vi "filter.insert.order.vi"(11 "filter.data in":T1 {"memory.command"."order.slot.value"."Quantity" format="%016x"; "memory.command"."order.slot.value"."OrderId" format="%016x"; "memory.command"."ticker.slot.value"."Symbol" format="%016x"; "Scratch"."OrderId" format="%016x"}) -> (3 "filter.data out":T1 {"memory.command"."order.slot.value"."Quantity" format="%016x"; "memory.command"."order.slot.value"."OrderId" format="%016x"; "memory.command"."ticker.slot.value"."Symbol" format="%016x"; "Scratch"."OrderId" format="%016x"})   [LabVIEW 2022 SP3]
uses:
  filter.data.ctl
  filter.states.ctl
  filter.debug.ctl
  filter.debug.slot.ctl
  filter.data.scratch.ctl
  arty/orderbook/orderbook.command.ctl
  arty/orderbook/orderbook.command.type.ctl
  filter.memory.command.ctl
  ticker.slot.ctl
  order.slot.ctl
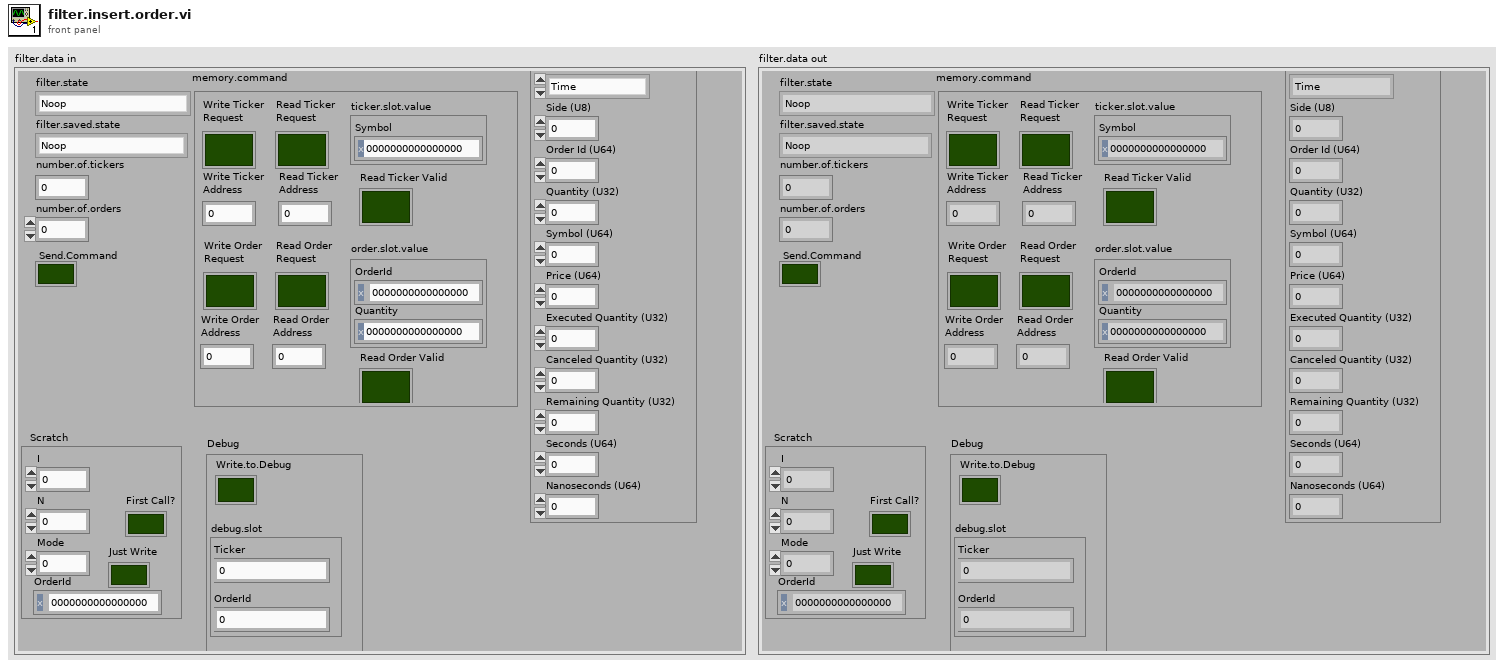
[diagram p1: front panel]
types:
  T1 = typedef "filter.data.ctl" = cluster{"filter.state":T2, "Debug":T3, "number.of.tickers":u32, "number.of.orders":u32, "filter.saved.state":T2, "Scratch":T5, "OrderBook.Command":T6, "Send.Command":bool, "memory.command":T8}
  T2 = typedef "filter.states.ctl" = enum16{"Noop", "Reset", "Debug", "Configuration", "Wait.for.Command", "Filter.Add", "Filter.Other", "Insert.Order", "Delete Order"}
  T3 = typedef "filter.debug.ctl" = cluster{"Write.to.Debug":bool, "debug.slot":T4}
  T4 = typedef "filter.debug.slot.ctl" = cluster{"Ticker":u64, "OrderId":u64}
  T5 = typedef "filter.data.scratch.ctl" = cluster{"I":u32, "N":u32, "Mode":u32, "OrderId":u64, "First Call?":bool, "Just Write":bool}
  T6 = typedef "orderbook.command.ctl" = cluster{"OrderBook Command.Type":T7, "Side (U8)":u8, "Order Id (U64)":u64, "Quantity (U32)":u32, "Symbol (U64)":u64, "Price (U64)":u64, "Executed Quantity (U32)":u32, "Canceled Quantity (U32)":u32, "Remaining Quantity (U32)":u32, "Seconds (U64)":u64, "Nanoseconds (U64)":u64}
  T7 = typedef "orderbook.command.type.ctl" = enum16{"Time", "AddOrder", "OrderExecuted", "OrderExecutedAtPrice", "ReduceSize", "ModifyOrder", "DeleteOrder", "Get.All.Orders", "Get.Top"}
  T8 = typedef "filter.memory.command.ctl" = cluster{"ticker.slot.value":T9, "order.slot.value":T10, "Write Ticker\nAddress":u32, "Write Ticker\nRequest":bool, "Read Ticker\nRequest":bool, "Read Ticker\nAddress":u32, "Read Ticker Valid":bool, "Write Order\nAddress":u32, "Write Order\nRequest":bool, "Read Order\nRequest":bool, "Read Order\nAddress":u32, "Read Order Valid":bool}
  T9 = typedef "ticker.slot.ctl" = cluster{"Symbol":u64}
  T10 = typedef "order.slot.ctl" = cluster{"OrderId":u64, "Quantity":u64}
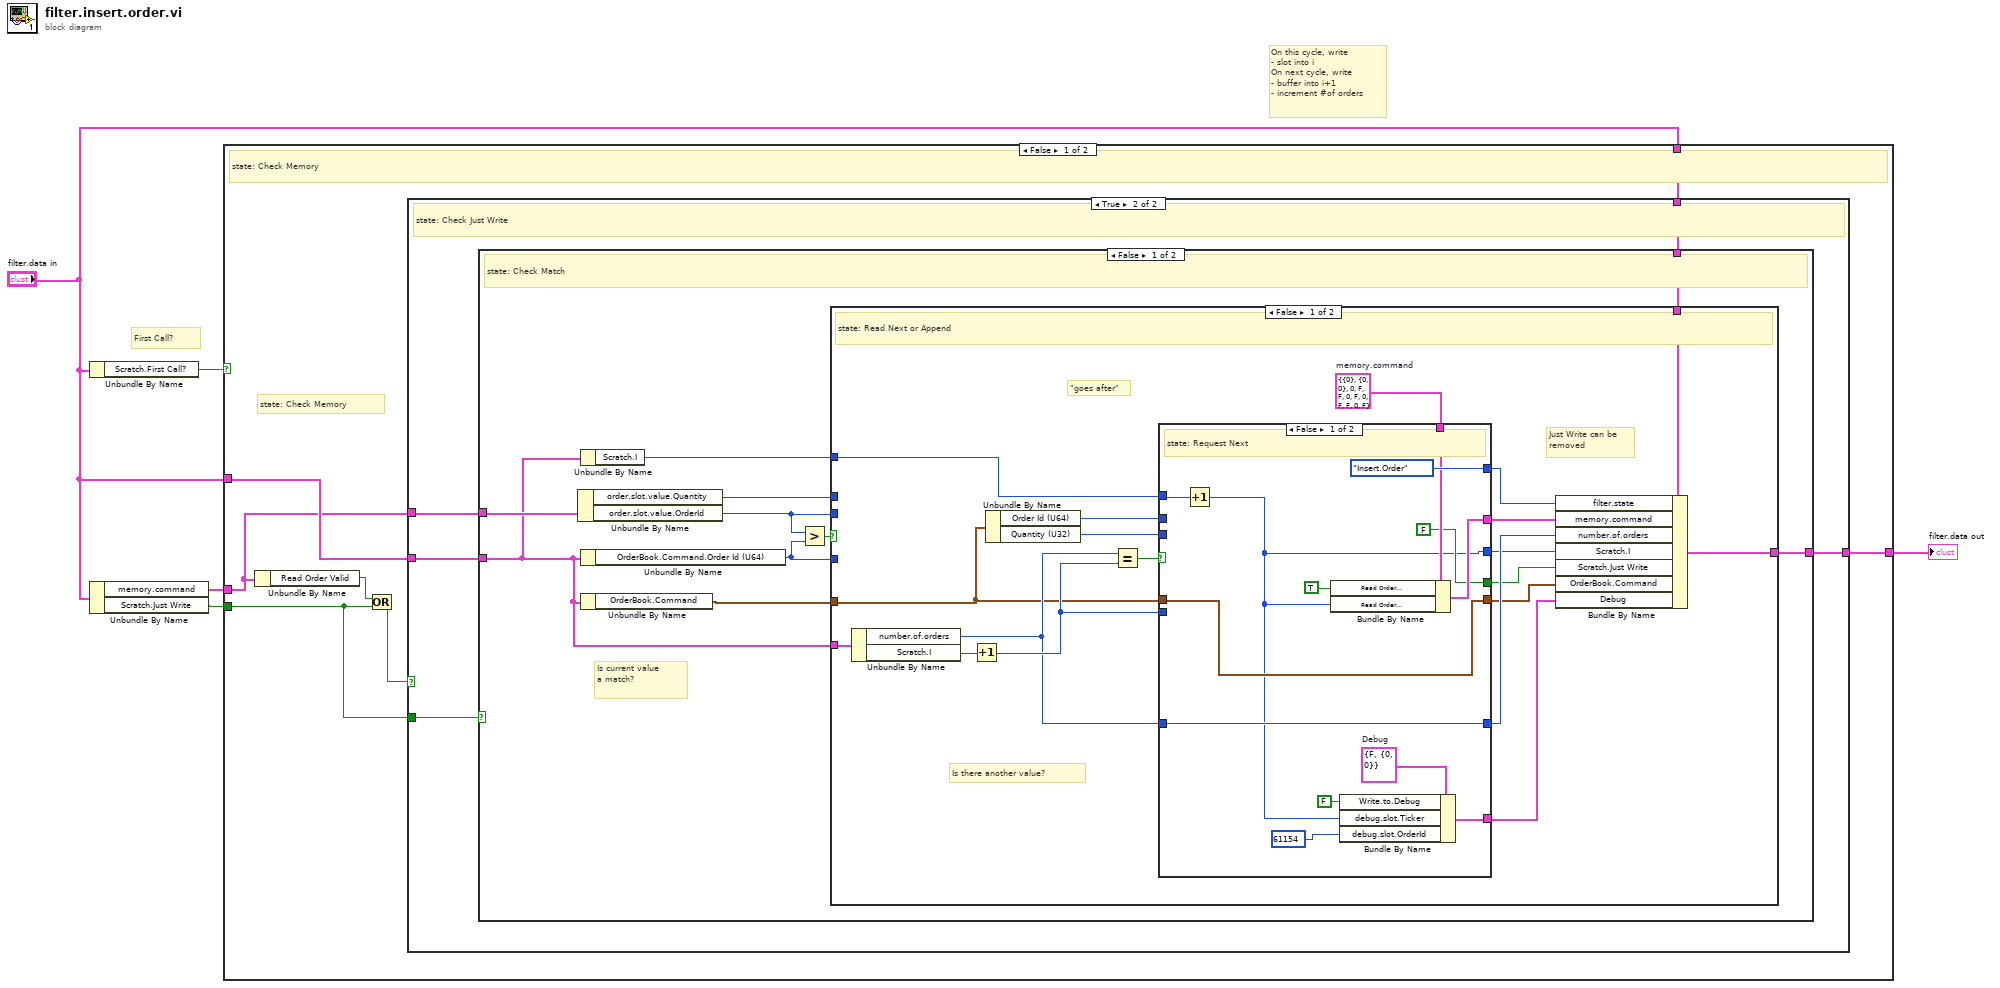
[diagram p0: block diagram]
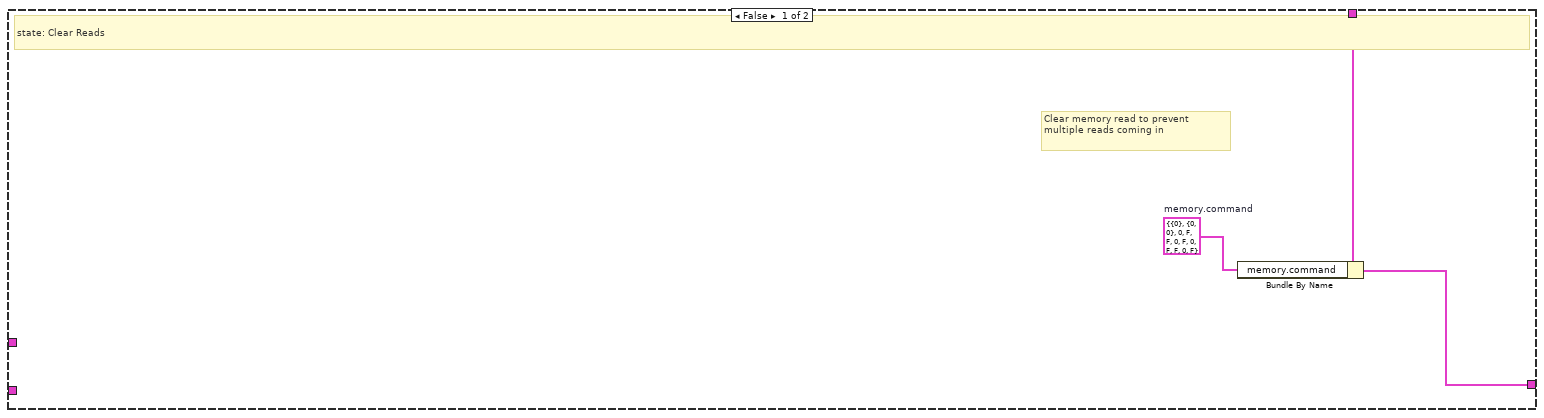
[diagram p2: hidden frame]
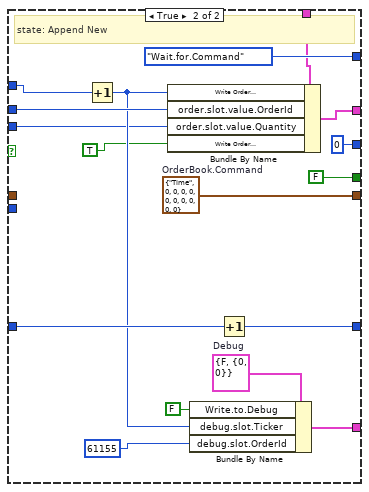
[diagram p3: hidden frame]
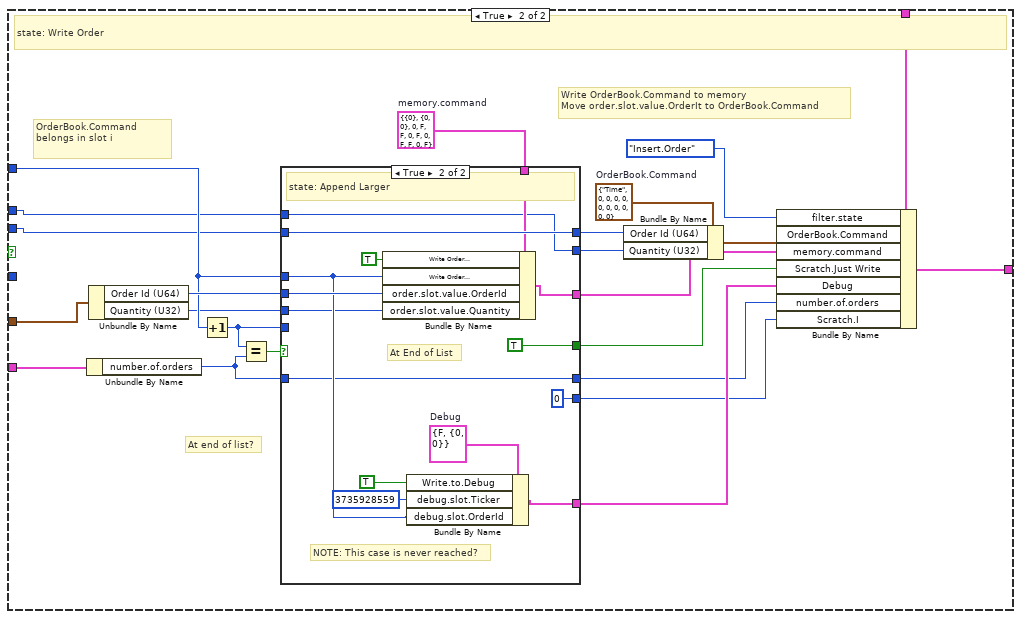
[diagram p4: hidden frame]
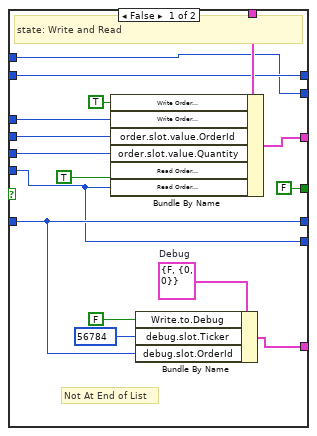
[diagram p5: hidden frame]
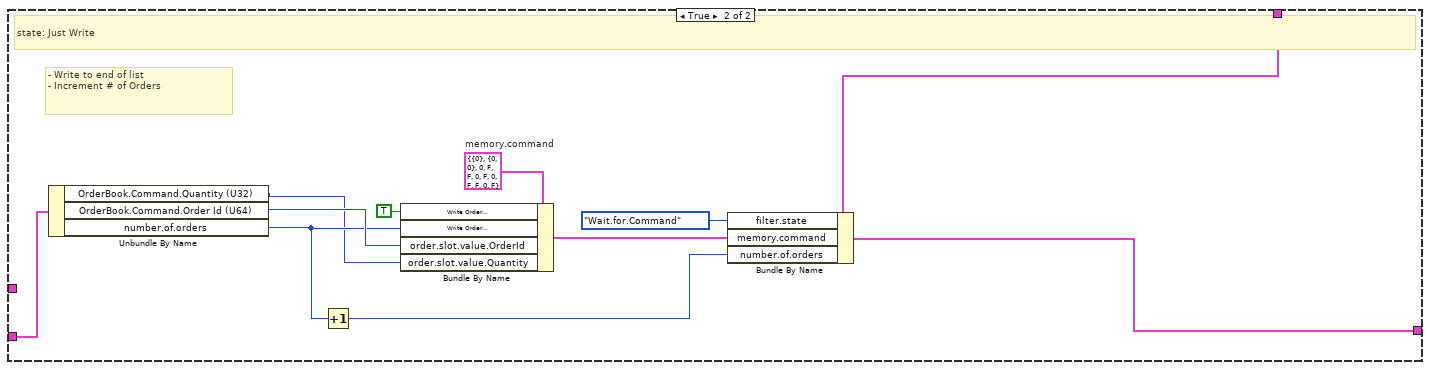
[diagram p6: hidden frame]
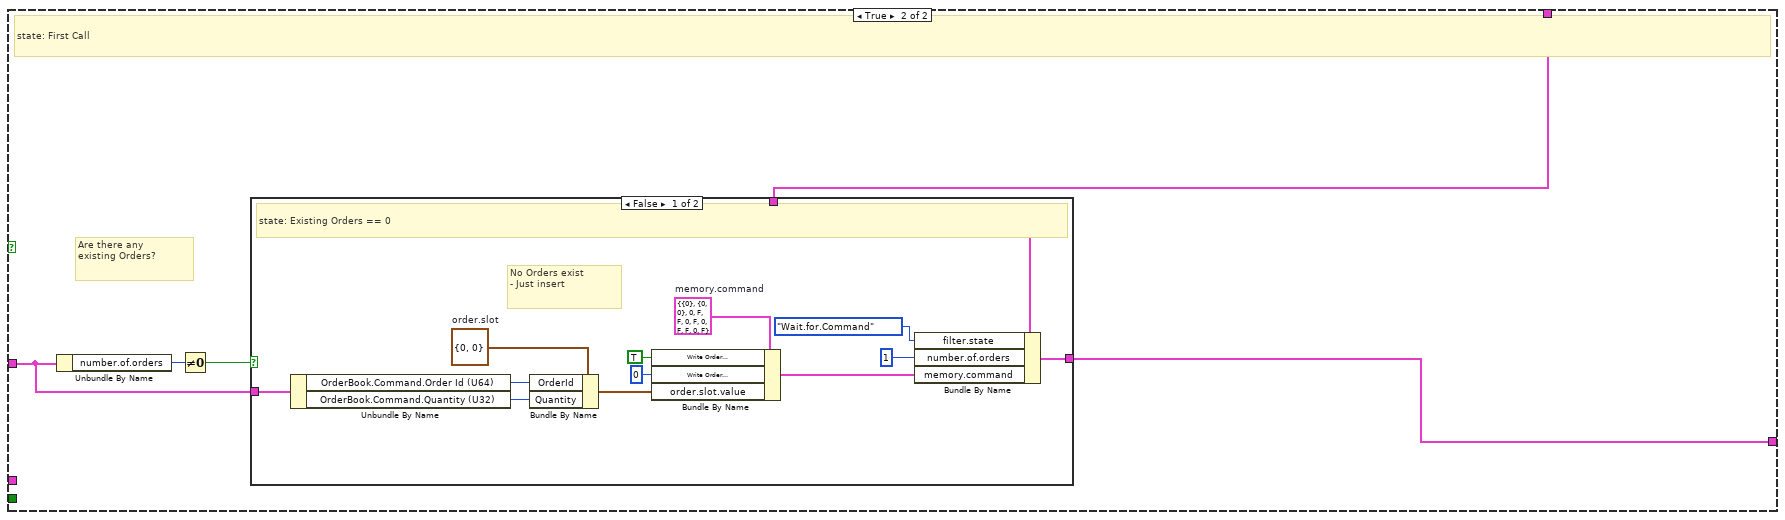
[diagram p7: hidden frame]
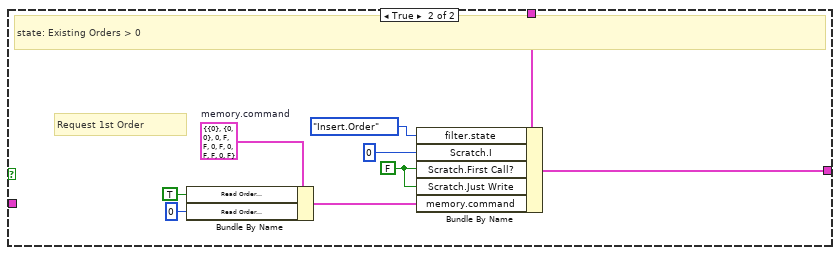
[diagram p8: hidden frame]
diagram:
  # "On this cycle, write\n- slot into i\nOn next cycle, write\n- buffer into i+1\n- increment #of orders"
  # "First Call?"
  n1 = Unbundle By Name("filter.data in") -> ("Scratch.First Call?"=w2:bool)
  n2 = Unbundle By Name("filter.data in") -> ("memory.command"=w4:T8, "Scratch.Just Write"=w1:bool)
  n3 = case shown="False" w2 {
    tunnel: "filter.data in" -> [w11 w147]
    tunnel: [w12 w145] -> w3
    tunnel: w4 -> [w9 _]
    tunnel: "filter.data in" -> [w10 w146]
    tunnel: w1 -> [w6 _]
    frame False {
      # "state: Check Memory"
      # "state: Check Memory"
      n4 = Unbundle By Name(w9) -> ("Read Order Valid"=w8:bool)
      n5 = Or(x=w8, y=w6) -> (x .or. y?=w7:bool)
      n6 = case shown="True" w7 {
        tunnel: [w13 w18] -> w12
        tunnel: w11 -> [w15 w19]
        tunnel: w10 -> [_ w17]
        tunnel: w9 -> [_ w20]
        tunnel: w6 -> [_ w16]
        frame False {
          w14 = T8 {"ticker.slot.value"={"Symbol"=0}, "order.slot.value"={"OrderId"=0, "Quantity"=0}, "Write Ticker\nAddress"=0, "Write Ticker\nRequest"=FALSE, "Read Ticker\nRequest"=FALSE, "Read Ticker\nAddress"=0, "Read Ticker Valid"=FALSE, "Write Order\nAddress"=0, "Write Order\nRequest"=FALSE, "Read Order\nRequest"=FALSE, "Read Order\nAddress"=0, "Read Order Valid"=FALSE}  # memory.command
          # "Clear memory read to prevent\nmultiple reads coming in"
          # "state: Clear Reads"
          n7 = Bundle By Name(cluster=w15, "memory.command"=w14) -> (w13:T1)
        }
        frame True {
          # "state: Check Just Write"
          n8 = case shown="False" w16 {
            tunnel: w20 -> [w30 _]
            tunnel: w19 -> [w28 w141]
            tunnel: [w27 w140] -> w18
            tunnel: w17 -> [w23 w138]
            frame False {
              # "Is current value\na match?"
              # "state: Check Match"
              n9 = Unbundle By Name(w30) -> ("order.slot.value.Quantity"=w21:u64, "order.slot.value.OrderId"=w25:u64)
              n10 = Unbundle By Name(w23) -> ("Scratch.I"=w22:u32)
              n11 = Unbundle By Name(w23) -> ("OrderBook.Command.Order Id (U64)"=w24:u64)
              n12 = Unbundle By Name(w23) -> ("OrderBook.Command"=w26:T6)
              n13 = Greater?(x=w25, y=w24) -> (0:w29:bool)
              n14 = case shown="False" w29 {
                tunnel: w28 -> [w48 w102]
                tunnel: [w49 w100] -> w27
                tunnel: w26 -> [w33 w95]
                tunnel: w23 -> [w47 w92]
                tunnel: w25 -> [_ w87]
                tunnel: w22 -> [w38 w93]
                tunnel: w24 -> [_ _]
                tunnel: w21 -> [_ w80]
                frame False {
                  w40 = T8 {"ticker.slot.value"={"Symbol"=0}, "order.slot.value"={"OrderId"=0, "Quantity"=0}, "Write Ticker\nAddress"=0, "Write Ticker\nRequest"=FALSE, "Read Ticker\nRequest"=FALSE, "Read Ticker\nAddress"=0, "Read Ticker Valid"=FALSE, "Write Order\nAddress"=0, "Write Order\nRequest"=FALSE, "Read Order\nRequest"=FALSE, "Read Order\nAddress"=0, "Read Order Valid"=FALSE}  # memory.command
                  # "Just Write can be\nremoved"
                  # "\"goes after\""
                  # "Is there another value?"
                  # "state: Read Next or Append"
                  n15 = Unbundle By Name(w47) -> ("number.of.orders"=w37:u32, "Scratch.I"=w46:u32)
                  n16 = Increment(x=w46) -> (x+1=w43:u32)
                  n17 = Unbundle By Name(w33) -> ("Order Id (U64)"=w39:u64, "Quantity (U32)"=w31:u32)
                  n18 = Equal?(x=w37, y=w43) -> (x = y?=w44:bool)
                  n19 = case shown="False" w44 {
                    tunnel: [w62 w76] -> w45
                    tunnel: w43 -> [_ _]
                    tunnel: [filter.states."Insert.Order" ("filter.state") filter.states."Wait.for.Command" ("filter.state")] -> w42
                    tunnel: [w58 w72] -> w41
                    tunnel: w40 -> [w59 w78]
                    tunnel: w39 -> [_ w77]
                    tunnel: w38 -> [w51 w75]
                    tunnel: w37 -> [w58 w74]
                    tunnel: [w50 u32 0] -> w36
                    tunnel: [FALSE ("Scratch.Just Write") FALSE ("Scratch.Just Write")] -> w35
                    tunnel: [w56 w70] -> w34
                    tunnel: w33 -> [w56 _]
                    tunnel: [w54 w68] -> w32
                    tunnel: w31 -> [_ w63]
                    frame False {
                      w55 = T3 {"Write.to.Debug"=FALSE, "debug.slot"={"Ticker"=0, "OrderId"=0}}  # Debug
                      # "state: Request Next"
                      n20 = Increment(x=w51) -> (x+1=w50:u32)
                      n21 = Bundle By Name(cluster=w59, "Read Order\nRequest"=TRUE ("Read.Request"), "Read Order\nAddress"=w50) -> (w62:T8)
                      n22 = Bundle By Name(cluster=w55, "Write.to.Debug"=FALSE, "debug.slot.Ticker"=w50, "debug.slot.OrderId"=u64 61154) -> (w54:T3)
                    }
                    frame True {
                      w69 = T3 {"Write.to.Debug"=FALSE, "debug.slot"={"Ticker"=0, "OrderId"=0}}  # Debug
                      w70 = T6 {"OrderBook Command.Type"=enum."Time", "Side (U8)"=0, "Order Id (U64)"=0, "Quantity (U32)"=0, "Symbol (U64)"=0, "Price (U64)"=0, "Executed Quantity (U32)"=0, "Canceled Quantity (U32)"=0, "Remaining Quantity (U32)"=0, "Seconds (U64)"=0, "Nanoseconds (U64)"=0}  # OrderBook.Command
                      # "state: Append New"
                      n23 = Increment(x=w75) -> (x+1=w65:u32)
                      n24 = Bundle By Name(cluster=w78, "Write Order\nAddress"=w65, "order.slot.value.OrderId"=w77, "order.slot.value.Quantity"=w63, "Write Order\nRequest"=TRUE ("Write Order\nRequest")) -> (w76:T8)
                      n25 = Bundle By Name(cluster=w69, "Write.to.Debug"=FALSE, "debug.slot.Ticker"=w65, "debug.slot.OrderId"=u64 61155) -> (w68:T3)
                      n26 = Increment(x=w74) -> (x+1=w72:u32)
                    }
                  }
                  n27 = Bundle By Name(cluster=w48, "filter.state"=w42, "memory.command"=w45, "number.of.orders"=w41, "Scratch.I"=w36, "Scratch.Just Write"=w35, "OrderBook.Command"=w34, "Debug"=w32) -> (w49:T1)
                }
                frame True {
                  w98 = T6 {"OrderBook Command.Type"=enum."Time", "Side (U8)"=0, "Order Id (U64)"=0, "Quantity (U32)"=0, "Symbol (U64)"=0, "Price (U64)"=0, "Executed Quantity (U32)"=0, "Canceled Quantity (U32)"=0, "Remaining Quantity (U32)"=0, "Seconds (U64)"=0, "Nanoseconds (U64)"=0}  # OrderBook.Command
                  w97 = T8 {"ticker.slot.value"={"Symbol"=0}, "order.slot.value"={"OrderId"=0, "Quantity"=0}, "Write Ticker\nAddress"=0, "Write Ticker\nRequest"=FALSE, "Read Ticker\nRequest"=FALSE, "Read Ticker\nAddress"=0, "Read Ticker Valid"=FALSE, "Write Order\nAddress"=0, "Write Order\nRequest"=FALSE, "Read Order\nRequest"=FALSE, "Read Order\nAddress"=0, "Read Order Valid"=FALSE}  # memory.command
                  # "At end of list?"
                  # "Write OrderBook.Command to memory\nMove order.slot.value.OrderIt to OrderBook.Command"
                  # "OrderBook.Command\nbelongs in slot i"
                  # "state: Write Order"
                  n28 = Unbundle By Name(w92) -> ("number.of.orders"=w84:u32)
                  n29 = Unbundle By Name(w95) -> ("Order Id (U64)"=w94:u64, "Quantity (U32)"=w82:u32)
                  n30 = Increment(x=w93) -> (x+1=w91:u32)
                  n31 = Equal?(x=w91, y=w84) -> (x = y?=w90:bool)
                  n32 = case shown="True" w90 {
                    tunnel: w97 -> [w118 w132]
                    tunnel: [w117 w131] -> w96
                    tunnel: w94 -> [w116 w130]
                    tunnel: w93 -> [w113 w123]
                    tunnel: w91 -> [w105 _]
                    tunnel: [w112 w133] -> w89
                    tunnel: w87 -> [w112 w133]
                    tunnel: [FALSE ("Scratch.Just Write") TRUE ("Scratch.Just Write")] -> w88
                    tunnel: [w107 w124] -> w86
                    tunnel: [w106 w122] -> w85
                    tunnel: w84 -> [w106 w122]
                    tunnel: [w105 u32 0] -> w83
                    tunnel: w82 -> [w104 w120]
                    tunnel: [w103 w119] -> w81
                    tunnel: w80 -> [w103 w119]
                    frame False {
                      w110 = T3 {"Write.to.Debug"=FALSE, "debug.slot"={"Ticker"=0, "OrderId"=0}}  # Debug
                      # "Not At End of List"
                      # "state: Write and Read"
                      n33 = Bundle By Name(cluster=w118, "Write Order\nRequest"=TRUE ("Write Order\nRequest"), "Write Order\nAddress"=w113, "order.slot.value.OrderId"=w116, "order.slot.value.Quantity"=w104, "Read Order\nRequest"=TRUE ("Read Order\nRequest"), "Read Order\nAddress"=w105) -> (w117:T8)
                      n34 = Bundle By Name(cluster=w110, "Write.to.Debug"=FALSE, "debug.slot.Ticker"=u64 56784, "debug.slot.OrderId"=w106) -> (w107:T3)
                    }
                    frame True {
                      w127 = T3 {"Write.to.Debug"=FALSE, "debug.slot"={"Ticker"=0, "OrderId"=0}}  # Debug
                      # "NOTE: This case is never reached?"
                      # "At End of List"
                      # "state: Append Larger"
                      n35 = Bundle By Name(cluster=w132, "Write Order\nRequest"=TRUE ("Write Order\nRequest"), "Write Order\nAddress"=w123, "order.slot.value.OrderId"=w130, "order.slot.value.Quantity"=w120) -> (w131:T8)
                      n36 = Bundle By Name(cluster=w127, "Write.to.Debug"=TRUE, "debug.slot.Ticker"=u64 3735928559, "debug.slot.OrderId"=w123) -> (w124:T3)
                    }
                  }
                  n37 = Bundle By Name(cluster=w98, "Order Id (U64)"=w89, "Quantity (U32)"=w81) -> (w99:T6)
                  n38 = Bundle By Name(cluster=w102, "filter.state"=filter.states."Insert.Order", "OrderBook.Command"=w99, "memory.command"=w96, "Scratch.Just Write"=w88, "Debug"=w86, "number.of.orders"=w85, "Scratch.I"=w83) -> (w100:T1)
                }
              }
            }
            frame True {
              w142 = T8 {"ticker.slot.value"={"Symbol"=0}, "order.slot.value"={"OrderId"=0, "Quantity"=0}, "Write Ticker\nAddress"=0, "Write Ticker\nRequest"=FALSE, "Read Ticker\nRequest"=FALSE, "Read Ticker\nAddress"=0, "Read Ticker Valid"=FALSE, "Write Order\nAddress"=0, "Write Order\nRequest"=FALSE, "Read Order\nRequest"=FALSE, "Read Order\nAddress"=0, "Read Order Valid"=FALSE}  # memory.command
              # "- Write to end of list\n- Increment # of Orders"
              # "state: Just Write"
              n39 = Unbundle By Name(w138) -> ("OrderBook.Command.Quantity (U32)"=w134:u32, "OrderBook.Command.Order Id (U64)"=w137:u64, "number.of.orders"=w135:u32)
              n40 = Increment(x=w135) -> (x+1=w136:u32)
              n41 = Bundle By Name(cluster=w142, "Write Order\nRequest"=TRUE ("Write Order\nRequest"), "Write Order\nAddress"=w135, "order.slot.value.OrderId"=w137, "order.slot.value.Quantity"=w134) -> (w139:T8)
              n42 = Bundle By Name(cluster=w141, "filter.state"=filter.states."Wait.for.Command", "memory.command"=w139, "number.of.orders"=w136) -> (w140:T1)
            }
          }
        }
      }
    }
    frame True {
      # "Are there any\nexisting Orders?"
      # "state: First Call"
      n43 = Unbundle By Name(w146) -> ("number.of.orders"=w149:u32)
      n44 = Not Equal To 0?(x=w149) -> (x != 0?=w148:bool)
      n45 = case shown="False" w148 {
        tunnel: w147 -> [w152 w166]
        tunnel: w146 -> [w153 _]
        tunnel: [w151 w165] -> w145
        frame False {
          w158 = T10 {"OrderId"=0, "Quantity"=0}  # order.slot
          w161 = T8 {"ticker.slot.value"={"Symbol"=0}, "order.slot.value"={"OrderId"=0, "Quantity"=0}, "Write Ticker\nAddress"=0, "Write Ticker\nRequest"=FALSE, "Read Ticker\nRequest"=FALSE, "Read Ticker\nAddress"=0, "Read Ticker Valid"=FALSE, "Write Order\nAddress"=0, "Write Order\nRequest"=FALSE, "Read Order\nRequest"=FALSE, "Read Order\nAddress"=0, "Read Order Valid"=FALSE}  # memory.command
          # "No Orders exist\n- Just insert"
          # "state: Existing Orders == 0"
          n46 = Unbundle By Name(w153) -> ("OrderBook.Command.Order Id (U64)"=w155:u64, "OrderBook.Command.Quantity (U32)"=w154:u32)
          n47 = Bundle By Name(cluster=w158, "OrderId"=w155, "Quantity"=w154) -> (w157:T10)
          n48 = Bundle By Name(cluster=w161, "Write Order\nRequest"=TRUE ("Read.Request"), "Write Order\nAddress"=u32 0 ("Write Order\nAddress"), "order.slot.value"=w157) -> (w150:T8)
          n49 = Bundle By Name(cluster=w152, "filter.state"=filter.states."Wait.for.Command", "number.of.orders"=u32 1, "memory.command"=w150) -> (w151:T1)
        }
        frame True {
          w163 = FALSE ("Scratch.First Call?")
          w171 = T8 {"ticker.slot.value"={"Symbol"=0}, "order.slot.value"={"OrderId"=0, "Quantity"=0}, "Write Ticker\nAddress"=0, "Write Ticker\nRequest"=FALSE, "Read Ticker\nRequest"=FALSE, "Read Ticker\nAddress"=0, "Read Ticker Valid"=FALSE, "Write Order\nAddress"=0, "Write Order\nRequest"=FALSE, "Read Order\nRequest"=FALSE, "Read Order\nAddress"=0, "Read Order Valid"=FALSE}  # memory.command
          # "Request 1st Order"
          # "state: Existing Orders > 0"
          n50 = Bundle By Name(cluster=w171, "Read Order\nRequest"=TRUE ("Read.Request"), "Read Order\nAddress"=u32 0 ("Read Order\nAddress")) -> (w164:T8)
          n51 = Bundle By Name(cluster=w166, "filter.state"=filter.states."Insert.Order", "Scratch.I"=u32 0, "Scratch.First Call?"=w163, "Scratch.Just Write"=w163, "memory.command"=w164) -> (w165:T1)
        }
      }
    }
  }
  "filter.data out" <- w3
